vi "33500b_adjust_output_level.vi"(8 "错误输入（无错误）":errorcluster, 9 "Amp(vpp)":dbl=1.0 format="%#_13g", 11 "Waveform Generator":refnum<visa-resource-name>) -> (0 "错误输出":errorcluster, 3 "Waveform Generator":refnum<visa-resource-name>)   [LabVIEW 2016]
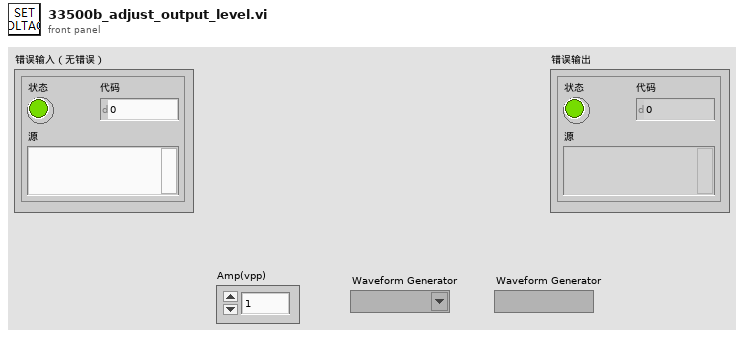
[diagram p1: front panel]
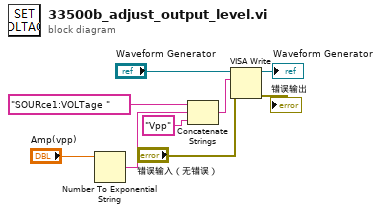
[diagram p0: block diagram]
diagram:
  n1 = Number To Exponential String(number="Amp(vpp)") -> (E-format string=w9:string)  [unwired: 3 in]
  n2 = Concatenate Strings("SOURce1:VOLTage " ("写入缓冲区"), w9, "Vpp" ("字符串")) -> (w5:string)
  n3 = VISA Write(VISA resource name="Waveform Generator", write buffer=w5, error in (no error)="错误输入（无错误）") -> (VISA resource name out=→"Waveform Generator":refnum<visa-resource-name>, error out=→"错误输出":errorcluster)  [unwired: 1 out]
